vi "PH_Watchdog.ProcCases.vi"(0 "i ref in":refnum<vi>, 1 "selector":string, 2 "Data":T1, 3 "call cluster":T2={"Object"="", "Selector"="", "CallType"=enum."synchronous", "Async Object"="", "Async Selector"="", "Data Descriptor"="", "Data"=[], "Error #"=0, "Expire"=0}, 5 "error in (no error)":errorcluster) -> (14 "i ref out":refnum<vi>, 17 "answer cluster":T2={"Object"="", "Selector"="", "CallType"=enum."synchronous", "Async Object"="", "Async Selector"="", "Data Descriptor"="", "Data"=[], "Error #"=0, "Expire"=0}, 19 "error out":errorcluster)   [LabVIEW 2014, in "PH_Watchdog.lvlib"]
doc: "This method is called by a process from within the default case in the event loop. The methods of a class that are linked to events will be called from THIS method. Add your code here."
uses:
  PH_Watchdog.lvlib
  CS_Core/CSSystem/CoreDefs/CoreDefs.call_type.ctl
  CS_Core/BaseProcess/BaseProcess.descriptor string definition.ctl
  CS_Core/CSSystem/CoreDefs/CoreDefs.rawDataType.ctl
  CS_Core/CSSystem/CoreLib/CoreLib.string 2 byte array.vi
  CS_Core/BaseProcess/BaseProcess.lvlib
  CS_Core/CSSystem/CoreLib/CoreLib.lvlib
  CS_Core/CAEObj/CAEObj.lvlib
  PH_Basics/PH_StatusHandler/PH_StatusHandler.lvlib
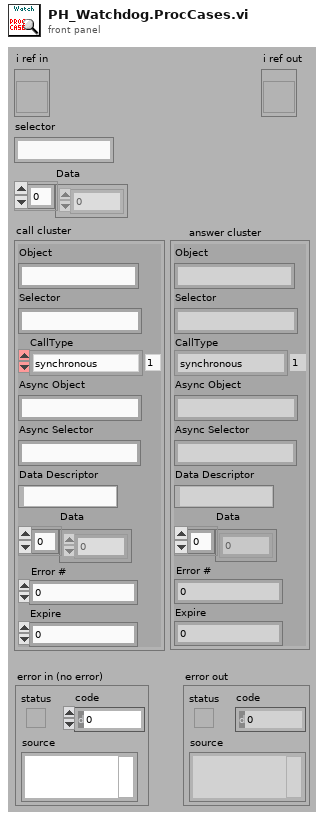
[diagram p1: front panel]
types:
  T1 = typedef "CoreDefs.rawDataType.ctl" = i8[]
  T2 = typedef "CoreDefs.call_type.ctl" = cluster{"Object":string, "Selector":string, "CallType":enum16{"simple", "synchronous", "asynchronous"}, "Async Object":string, "Async Selector":string, "Data Descriptor":T3, "Data":T1, "Error #":i32, "Expire":u32}
  T3 = typedef "BaseProcess.lvlib/BaseProcess.descriptor string definition.ctl" = string
  T4 = typedef "PH_Watchdog.lvlib/PH_Watchdog.i attribute.ctl" = cluster{"GUI Refs":cluster{"All":refnum<vi>, "Failures":refnum<vi>, "Alarms":refnum<vi>, "no info, but linked":refnum<vi>}, "All":T5[]}
  T5 = typedef "PH_Watchdog.lvlib/PH_Watchdog.Dataset.ctl" = cluster{"Instance":string, "Class":string, "Status":T6, "no Link":bool}
  T6 = typedef "PH_StatusHandler.lvlib/PH_StatusHandler.Status.ctl" = i16
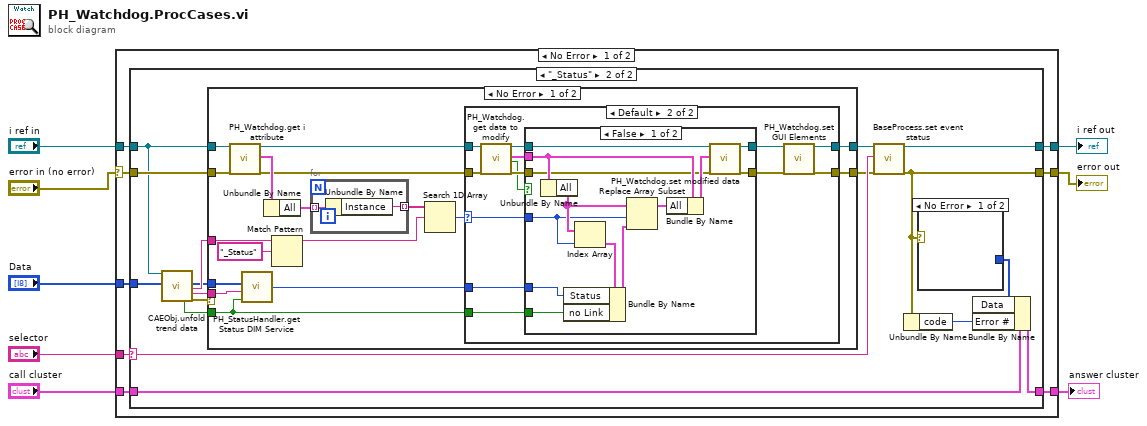
[diagram p0: block diagram]
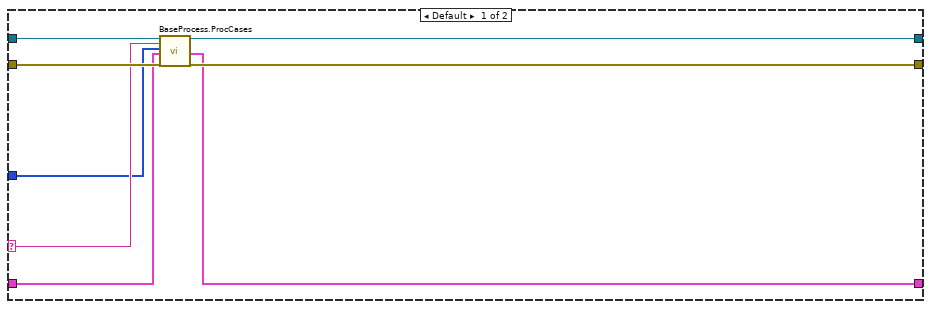
[diagram p2: hidden frame]
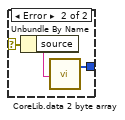
[diagram p6: hidden frame]
diagram:
  n1 = case shown="No Error" "error in (no error)" {
    selector: "error in (no error)" -> [w9 w97]
    tunnel: "selector" -> [w16 _]
    tunnel: [w15 w96] -> w7
    tunnel: "call cluster" -> [w14 w96]
    tunnel: "i ref in" -> [w13 w98]
    tunnel: [w12 w98] -> w4
    tunnel: [w11 w97] -> w3
    tunnel: "Data" -> [w10 _]
    frame No Error {
      n2 = case shown="\"_Status\"" w16 {
        selector: w16 -> [w19 w37]
        tunnel: w10 -> [w17 w28]
        tunnel: w13 -> [w18 w27]
        tunnel: [w24 w39] -> w12
        tunnel: w14 -> [w20 w36]
        tunnel: [w21 w35] -> w15
        tunnel: w9 -> [w23 w31]
        tunnel: [w22 w38] -> w11
        frame Default {
          n3 = call "BaseProcess.ProcCases.vi"("i ref in"=w18, "selector"=w19, "Data"=w17, "call cluster"=w20, "error in (no error)"=w23) -> ("i ref out"=w24:refnum<vi>, "answer cluster"=w21:T2, "error out"=w22:errorcluster)  [unwired: 12 in]
        }
        frame "_Status" {
          n4 = call "CAEObj.unfold trend data.vi"("i ref in"=w27, "raw trend data"=w28) -> ("no link"=w33:bool, "data"=w26:i8[], "serviceName"=w32:string, "typeDescriptor"=w25:string, "error out"=w34:errorcluster)  [unwired: 9 in, 4 out]
          n5 = case shown="No Error" w34 {
            tunnel: [w55 w92] -> w30
            tunnel: w27 -> [w53 w92]
            tunnel: w31 -> [w58 w91]
            tunnel: w26 -> [w52 _]
            tunnel: w33 -> [w43 _]
            tunnel: w32 -> [w50 _]
            tunnel: [w54 w91] -> w29
            tunnel: w25 -> [w51 _]
            frame No Error {
              n6 = call "PH_Watchdog.get i attribute.vi"("i ref in"=w53, "error in (no error)"=w58) -> ("i ref out"=w56:refnum<vi>, "i attribute"=w57:T4, "error out"=w44:errorcluster)  [unwired: 15 in]
              n7 = call "PH_StatusHandler.get Status DIM Service.vi"("no link"=w43, "typeDescriptor"=w51, "data"=w52) -> ("Status"=w42:T6)  [unwired: 1 in]
              n8 = Unbundle By Name(w57) -> ("All"=w48:T5[])
              n9 = Match Pattern(string=w50, regular expression="_Status") -> (before substring=w46:string)  [unwired: 1 in, 3 out]
              n10 = for {
                tunnel: w48 -> [w60] mode=indexing
                tunnel: [w59] -> w47 mode=indexing
                n11 = Unbundle By Name(w60) -> ("Instance"=w59:string)
              }
              n12 = Search 1D Array(1D array=w47, element=w46) -> (index of element=w45:i32)  [unwired: 1 in]
              n13 = case shown="Default" w45 {
                selector: w45 -> [_ w68]
                tunnel: w56 -> [w62 w75]
                tunnel: w44 -> [w61 w74]
                tunnel: [w62 w63] -> w55
                tunnel: [w61 w65] -> w54
                tunnel: w43 -> [_ w67]
                tunnel: w42 -> [_ w66]
                frame -1 {
                }
                frame Default {
                  n14 = call "PH_Watchdog.get data to modify.vi"("i ref in"=w75, "error in (no error)"=w74) -> ("i ref out"=w73:refnum<vi>, "i attribute"=w70:T4, "timed out"=w69:bool, "error out"=w72:errorcluster)  [unwired: 14 in]
                  n15 = case shown="False" w69 {
                    tunnel: w73 -> [w88 w90]
                    tunnel: [w87 w90] -> w64
                    tunnel: w72 -> [w78 w89]
                    tunnel: [w86 w89] -> w71
                    tunnel: w70 -> [w84 _]
                    tunnel: w68 -> [w82 _]
                    tunnel: w67 -> [w77 _]
                    tunnel: w66 -> [w76 _]
                    frame False {
                      n16 = Unbundle By Name(w84) -> ("All"=w83:T5[])
                      n17 = Index Array(array=w83, index=w82) -> (element=w80:T5)
                      n18 = Bundle By Name(cluster=w80, "Status"=w76, "no Link"=w77) -> (w79:T5)
                      n19 = Replace Array Subset(array=w83, new element=w79, index=w82) -> (w81:T5[])
                      n20 = Bundle By Name(cluster=w84, "All"=w81) -> (w85:T4)
                      n21 = call "PH_Watchdog.set modified data.vi"("i ref in"=w88, "i attribute"=w85, "error in (no error)"=w78) -> ("i ref out"=w87:refnum<vi>, "error out"=w86:errorcluster)  [unwired: 15 in]
                    }
                    frame True {
                    }
                  }
                  n22 = call "PH_Watchdog.set GUI Elements.vi"("VI in"=w64, "error in"=w71) -> ("VI out"=w63:refnum<vi>, "error out"=w65:errorcluster)  [unwired: 16 in]
                }
              }
            }
            frame Error {
            }
          }
          n23 = call "BaseProcess.set event status.vi"("i ref in"=w30, "EventStatus"=w37, "error in (no error)"=w29) -> ("i ref out"=w39:refnum<vi>, "error out"=w38:errorcluster)  [unwired: 14 in, 1 out]
          n24 = Unbundle By Name(w38) -> ("code"=w41:i32)
          n25 = case shown="No Error" w38 {
            selector: w38 -> [_ w95]
            tunnel: [_ w93] -> w40
            frame No Error {
            }
            frame Error {
              n26 = Unbundle By Name(w95) -> ("source"=w94:string)
              n27 = call-poly "CoreLib.data 2 byte array.vi"("string"=w94) -> ("byteArray out"=w93:T1)  [unwired: 18 in]
            }
          }
          n28 = Bundle By Name(cluster=w36, "Data"=w40, "Error #"=w41) -> (w35:T2)
        }
      }
    }
    frame Error {
    }
  }
  "answer cluster" <- w7
  "i ref out" <- w4
  "error out" <- w3
